vi "Exponents--constant.vi"() -> (1 "exponent":dbl[](array[numeric]))   [LabVIEW 2018, in "Resistance Value.lvlib"]
doc: "Provides the exponent array used to determine the numerical multiplier value from the resistor multiplier color.\n\nThe array contains the exponent values corresponding to the resistor color code:\n\n[-2, -1, 0, 1, 2, 3, 4, 5, 6, 7, 8, 9]\n\nThe index of each element corresponds to the value of the Multiplier Color Enum.\n\nThe array is used by the multiplier conversion VI to obtain the exponent associated with the selected multiplier color."
uses:
  Resistance Value.lvlib
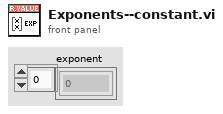
[diagram p1: front panel]
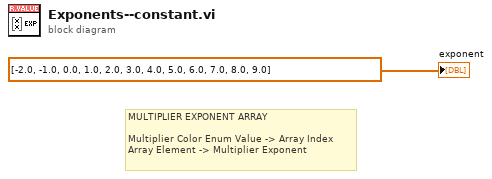
[diagram p0: block diagram]
diagram:
  # "MULTIPLIER EXPONENT ARRAY\n\nMultiplier Color Enum Value -> Array Index\nArray Element -> Multiplier Exponent"
  "exponent" <- dbl[] [-2.0, -1.0, 0.0, 1.0, 2.0, 3.0, 4.0, 5.0, 6.0, 7.0, 8.0, 9.0]
